vi "unCover.vi"(8 "error in (no error)":errorcluster, 11 "Cell in":refnum<class "Cell.lvclass">) -> (0 "error out":errorcluster, 2 "BOOOOOOOM!":bool, 3 "Cell out":refnum<class "Cell.lvclass">)   [LabVIEW 2014, in "Cell.lvclass"]
uses:
  Cell.lvclass
  Cell.lvclass/Cell.ctl
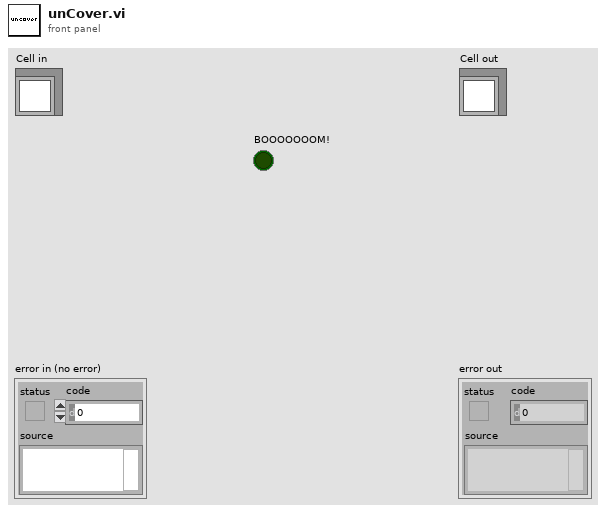
[diagram p1: front panel]
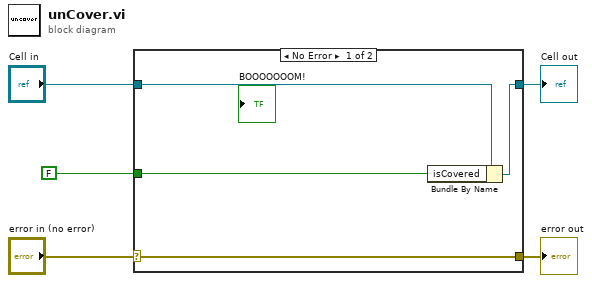
[diagram p0: block diagram]
diagram:
  n1 = case shown="No Error" "error in (no error)" {
    selector: "error in (no error)" -> [w9 w10]
    tunnel: [w9 w10] -> w4
    tunnel: [w7 w11] -> w2
    tunnel: "Cell in" -> [w8 w11]
    tunnel: FALSE ("isCovered") -> [w6 _]
    frame No Error {
      n2 = Bundle By Name(cluster=w8, "isCovered"=w6) -> (w7:refnum<class "Cell.lvclass">)
    }
    frame Error {
    }
  }
  "error out" <- w4
  "Cell out" <- w2
